vi "Read_Power.vi"(8 "error in (no error)":errorcluster={"status"=FALSE, "code"=1073676294, "source"="VISA Read in Read Current in Arms.vi->LV2017CP.vi"}, 11 "VISA Refnum in":refnum<visa-resource-name>="COM8") -> (0 "error out":errorcluster={"status"=FALSE, "code"=1073676294, "source"="VISA Read in Read I_q in Arms.vi->LV2017CP.vi"}, 2 "read buffer":string, 3 "VISA Refnum out":refnum<visa-resource-name>="COM8")   [LabVIEW 2016]
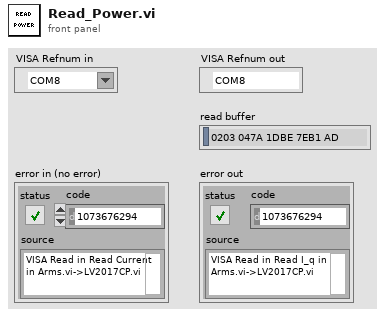
[diagram p1: front panel]
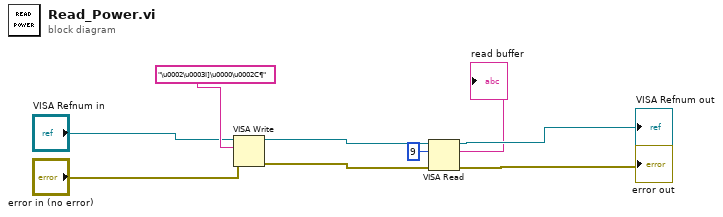
[diagram p0: block diagram]
diagram:
  n1 = VISA Write(VISA resource name="VISA Refnum in", write buffer="\u0002\u0003I]\u0000\u0002C¶", error in (no error)="error in (no error)") -> (VISA resource name out=w3:refnum<visa-resource-name>, error out=w4:errorcluster)  [unwired: 1 out]
  n2 = VISA Read(VISA resource name=w3, byte count=u32 9, error in (no error)=w4) -> (VISA resource name out=→"VISA Refnum out":refnum<visa-resource-name>, read buffer=→"read buffer":string, error out=→"error out":errorcluster)  [unwired: 1 out]
